vi "例5.14  生成一段正弦波形.vi"() -> ()   [LabVIEW 2017]
panel:
  in  "点数/周期":dbl
  in  "周期数":dbl
  in  "频率":dbl
  in  "初相位":dbl
  in  "幅值":dbl
  out "波形图":waveform(dbl)(graph)
  out "输出波形":waveform(dbl)
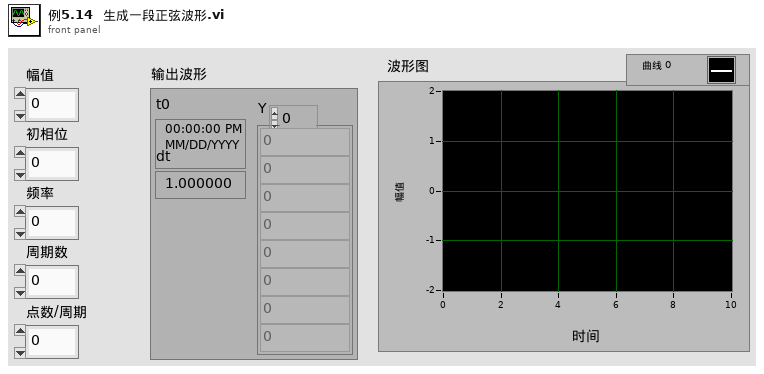
[diagram p1: front panel]
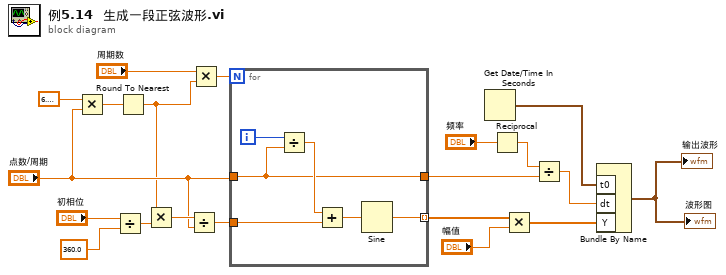
[diagram p0: block diagram]
diagram:
  n1 = Multiply(x=6.283185307179586, y="点数/周期") -> (x*y=w8:dbl)
  n2 = Divide(x="初相位", y=360.0) -> (x/y=w11:dbl)
  n3 = Round To Nearest(number=w8) -> (nearest integer value=w2:dbl)
  n4 = Multiply(x=w2, y=w11) -> (x*y=w6:dbl)
  n5 = Divide(x=w6, y="点数/周期") -> (x/y=w5:dbl)
  n6 = Multiply(x="周期数", y=w2) -> (x*y=w7:dbl)
  n7 = for {
    N: w7 -> [_]
    tunnel: [w26] -> w19 mode=indexing
    tunnel: [w23] -> w15
    tunnel: "点数/周期" -> [w23]
    tunnel: w5 -> [w21]
    i -> [w25]
    n8 = Divide(x=w25, y=w23) -> (x/y=w24:dbl)
    n9 = Add(x=w24, y=w21) -> (x+y=w22:dbl)
    n10 = Sine(x=w22) -> (sin(x)=w26:dbl)
  }
  n11 = Get Date/Time In Seconds() -> (seconds since 1Jan1904=w1:timestamp)
  n12 = Reciprocal(x="频率") -> (1/x=w16:dbl)
  n13 = Multiply(x=w19, y="幅值") -> (x*y=w10:dbl[])
  n14 = Divide(x=w16, y=w15) -> (x/y=w14:dbl)
  n15 = Bundle By Name("t0"=w1, "dt"=w14, "Y"=w10) -> (→"输出波形" →"波形图":waveform(dbl))  [unwired: 1 in]
